vi "Validate if event is selected.vi"(11 "Tree Selection":string) -> (0 "Selection is Main.vi":bool, 1 "Selection is Module":bool, 2 "Selection is a Broadcast?":bool, 3 "Selection is an Event?":bool)   [LabVIEW 2019, in "Panther Dashboard.lvlib"]
uses:
  Panther Dashboard.lvlib
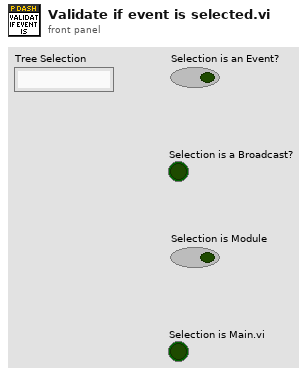
[diagram p1: front panel]
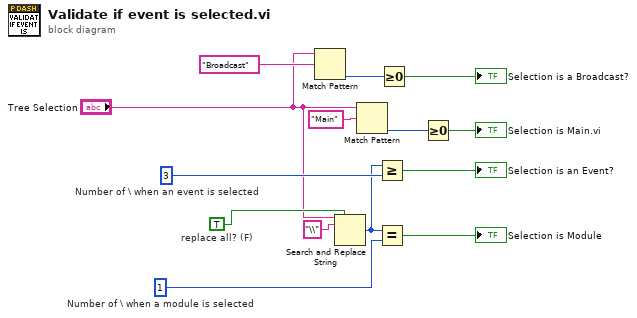
[diagram p0: block diagram]
diagram:
  w5 = 1  # Number of \ when a module is selected
  w13 = 3  # Number of \ when an event is selected
  w11 = TRUE  # replace all? (F)
  n1 = Match Pattern(string="Tree Selection", regular expression="Broadcast") -> (offset past match=w9:i32)  [unwired: 1 in, 3 out]
  n2 = Search and Replace String(replace all?=w11, input string="Tree Selection", search string="\\") -> (number of replacements=w7:i32)  [unwired: 5 in, 3 out]
  n3 = Match Pattern(string="Tree Selection", regular expression="Main") -> (offset past match=w2:i32)  [unwired: 1 in, 3 out]
  n4 = Greater Or Equal?(x=w7, y=w13) -> (x >= y?=→"Selection is an Event?":bool)
  n5 = Equal?(x=w7, y=w5) -> (x = y?=→"Selection is Module":bool)
  n6 = Greater Or Equal To 0?(x=w9) -> (x >= 0?=→"Selection is a Broadcast?":bool)
  n7 = Greater Or Equal To 0?(x=w2) -> (x >= 0?=→"Selection is Main.vi":bool)
